vi "Last Ack Creator.vi"(7 "Sender":refnum<class "Sender.lvclass">, 10 "jettl":refnum<class "jettl.lvclass">, 11 "Last Ack Creator in":refnum<class "Last Ack Creator.lvclass">) -> (3 "Last Ack Creator out":refnum<class "Last Ack Creator.lvclass">)   [LabVIEW 2021, in "jettl.lvlib" / "Last Ack Creator Msg Strategy.lvlib" / "Last Ack Creator.lvclass"]
uses:
  Last Ack Creator.lvclass
  jettl/jettl.lvclass
  Sender/Sender/Sender.lvclass
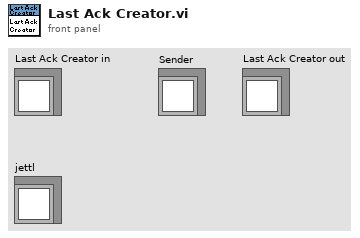
[diagram p1: front panel]
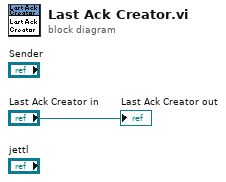
[diagram p0: block diagram]
diagram:
  "Last Ack Creator out" <- "Last Ack Creator in"
